vi "Script RPC Client VI.vi"(6 "rpc method parameters":T1, 7 "owning library":refnum<vi>, 8 "error in (no error)":errorcluster, 9 "rpc service name":string, 10 "owning folder":refnum<vi>, 11 "template project item":refnum<vi>) -> (0 "error out":errorcluster)   [LabVIEW 2019, in "gRPC Template Creation Utility.lvlib"]
uses:
  gRPC Template Creation Utility.lvlib
  TypeDefs/RPC Method Parameters.ctl
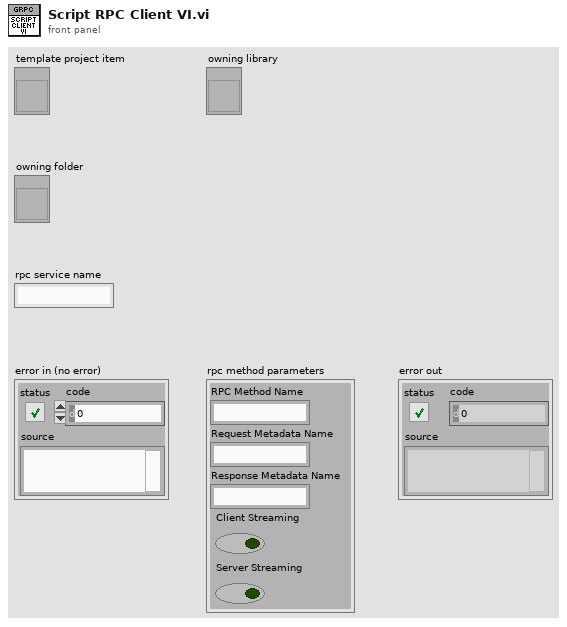
[diagram p1: front panel]
types:
  T1 = typedef "gRPC Template Creation Utility.lvlib/RPC Method Parameters.ctl" = cluster{"RPC Method Name":string, "Request Metadata Name":string, "Response Metadata Name":string, "Client Streaming":bool, "Server Streaming":bool}
  T2 = enum32{"invalid VI type", "Standard VI", "Control VI", "Global VI", "Polymorphic VI", "Configuration VI", "SubSystem", "Facade VI", "Method VI"}
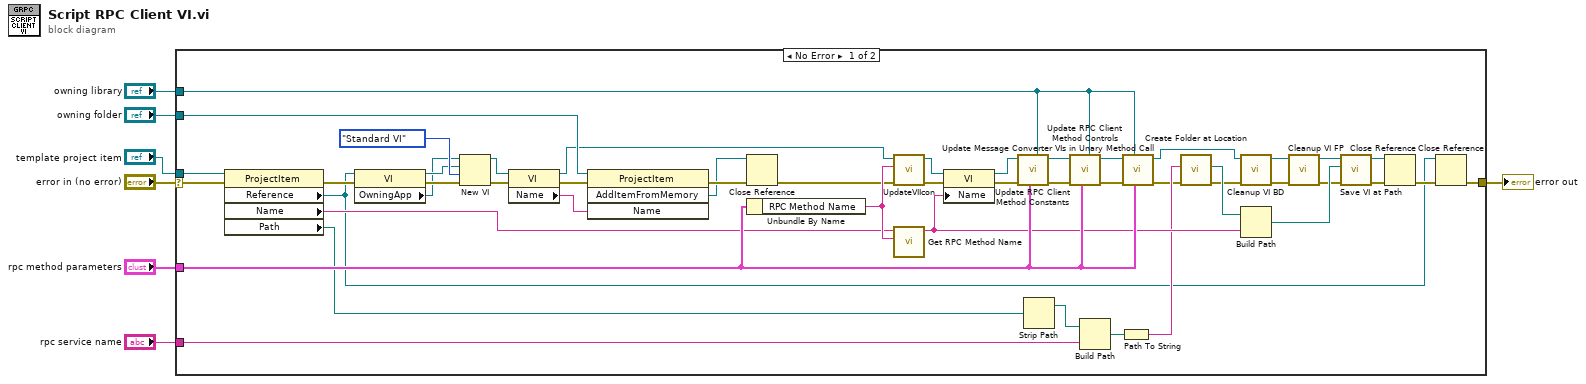
[diagram p0: block diagram]
diagram:
  n1 = case shown="No Error" "error in (no error)" {
    selector: "error in (no error)" -> [w28 w56]
    tunnel: "rpc method parameters" -> [w55 _]
    tunnel: "owning library" -> [w54 _]
    tunnel: [w9 w56] -> w5
    tunnel: "rpc service name" -> [w42 _]
    tunnel: "owning folder" -> [w40 _]
    tunnel: "template project item" -> [w31 _]
    frame No Error {
      n2 = property class="ProjectItem"(reference=w31, error in=w28) -> (error out=w14:errorcluster, "Reference"=w8:refnum<vi>, "Name"=w30:string, "Path"=w29:path)  [unwired: 1 out]
      n3 = property class="VI"(reference=w8, error in=w14) -> (reference out=w12:refnum<vi>, error out=w13:errorcluster, "OwningApp"=w11:refnum<vi>)
      n4 = New VI(8:w13, 9:T2."Standard VI" ("vi type (standard vi)"), 10:w12, 11:w11) -> (0:w26:errorcluster, 3:w27:refnum<vi>)  [unwired: 3 out]
      n5 = property class="VI"(reference=w27, error in=w26) -> (reference out=w25:refnum<vi>, error out=w34:errorcluster, "Name"=w32:string)
      n6 = invoke class="ProjectItem" method="AddItemFromMemory"(reference=w40, error in=w34, "Name"=w32) -> (error out=w39:errorcluster, "AddItemFromMemory"=w38:refnum<vi>)  [unwired: 1 in, 2 out]
      n7 = Close Reference(reference=w38, error in (no error)=w39) -> (error out=w22:errorcluster)
      n8 = Unbundle By Name(w55) -> ("RPC Method Name"=w51:string)
      n9 = call "UpdateVIIcon.vi"("error in (no error)"=w22, "Method Name"=w51, "VI in"=w25) -> ("error out"=w23:errorcluster, "VI out"=w24:refnum<vi>)  [unwired: 7 in]
      n10 = call "Get RPC Method Name.vi"("RPC Method Name"=w51, "Template VI Name"=w30) -> ("RPC VI Name"=w50:string)  [unwired: 8 in, 1 out]
      n11 = property class="VI"(reference=w24, error in=w23, "Name"=w50) -> (reference out=w48:refnum<vi>, error out=w46:errorcluster)
      n12 = call "Update RPC Client Method Constants.vi"("Library"=w54, "RPC Method Parameters"=w55, "error in (no error)"=w46, "VI in"=w48) -> ("error out"=w47:errorcluster, "VI out"=w49:refnum<vi>)  [unwired: 6 in]
      n13 = Strip Path(path=w29) -> (stripped path=w41:path)  [unwired: 1 out]
      n14 = call "Update RPC Client Method Controls.vi"("Library"=w54, "RPC Method Parameters"=w55, "error in (no error)"=w47, "VI in"=w49) -> ("error out"=w53:errorcluster, "VI out"=w52:refnum<vi>)  [unwired: 6 in]
      n15 = Build Path(base path=w41, name or relative path=w42) -> (appended path=w43:path)
      n16 = Path To String(path=w43) -> (string=w44:string)
      n17 = call "Update Message Converter VIs in Unary Method Call.vi"("RPC Method Parameters"=w55, "Library"=w54, "error in (no error)"=w53, "VI in"=w52) -> ("error out"=w21:errorcluster, "VI out"=w18:refnum<vi>)  [unwired: 6 in]
      n18 = call "Create Folder at Location.vi"("Error In"=w21, "Path"=w44) -> ("Error Out"=w16:errorcluster, "Full path out"=w45:path)  [unwired: 7 in, 1 out]
      n19 = call "Cleanup VI BD.vi"("error in (no error)"=w16, "VI in"=w18) -> ("error out"=w20:errorcluster, "VI out"=w19:refnum<vi>)  [unwired: 8 in]
      n20 = Build Path(base path=w45, name or relative path=w50) -> (appended path=w35:path)
      n21 = call "Cleanup VI FP.vi"("error in"=w20, "vi in"=w19) -> ("error out"=w15:errorcluster, "vi out"=w17:refnum<vi>)  [unwired: 8 in]
      n22 = call "Save VI at Path.vi"("error in (no error)"=w15, "Path"=w35, "VI in"=w17) -> ("error out"=w36:errorcluster, "VI out"=w37:refnum<vi>)  [unwired: 6 in, 1 out]
      n23 = Close Reference(reference=w37, error in (no error)=w36) -> (error out=w10:errorcluster)
      n24 = Close Reference(reference=w8, error in (no error)=w10) -> (error out=w9:errorcluster)
    }
    frame Error {
    }
  }
  "error out" <- w5
